vi "Test Selection.vi"() -> (0 "error out":errorcluster, 3 "Test Selected":string(combo))   [LabVIEW 2023, in "HardwareAbstractionLayer_LVOOP.lvlib" / "Report.lvclass"]
uses:
  Report.lvclass
panel:
  in  "Cancel":bool
  in  "Contionus Test":bool
  in  "New Test":bool
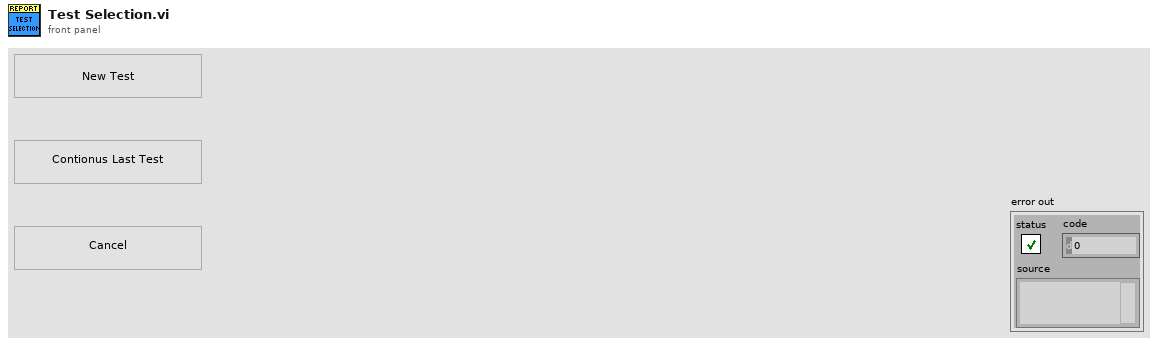
[diagram p1: front panel]
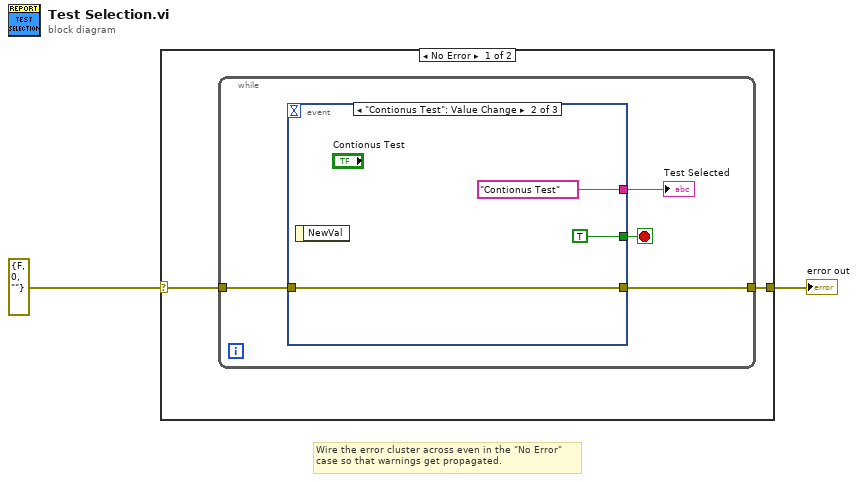
[diagram p0: block diagram]
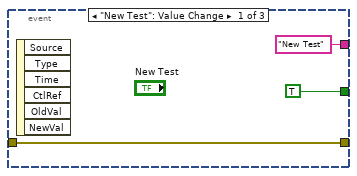
[diagram p2: hidden frame]
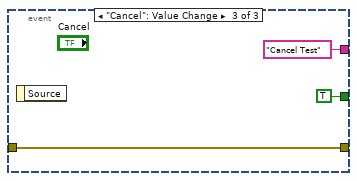
[diagram p3: hidden frame]
diagram:
  # "Wire the error cluster across even in the \"No Error\"\ncase so that warnings get propagated."
  n1 = case shown="No Error" errorcluster {"status"=FALSE, "code"=0, "source"=""} ("error in (no error)") {
    selector: errorcluster {"status"=FALSE, "code"=0, "source"=""} ("error in (no error)") -> [w4 w18]
    tunnel: [w3 w18] -> w2
    frame No Error {
      n2 = while {
        tunnel: w4 -> [w7]
        tunnel: [w6] -> w3
        stop <- w8 stop-if-true
        n3 = event shown="[1] \"Contionus Test\": Value Change" {
          selector: _ -> [_ _ _]
          dyn-events: _ -> [_ _ _]
          timeout: _ -> [_ _ _]
          tunnel: [TRUE TRUE TRUE] -> w8
          tunnel: w7 -> [w10 w13 w17]
          tunnel: [w10 w13 w17] -> w6
          tunnel: ["New Test" ("Test Selected") "Contionus Test" ("Test Selected") "Cancel Test" ("Test Selected")] -> w5
          event "New Test": Value Change {
            n4 = event-data() -> ()  [unwired: 1 in, 6 out]
          }
          event "Contionus Test": Value Change {
            n5 = event-data() -> ()  [unwired: 1 in, 1 out]
          }
          event "Cancel": Value Change {
            n6 = event-data() -> ()  [unwired: 1 in, 1 out]
          }
        }
        "Test Selected" <- w5
      }
    }
    frame Error {
    }
  }
  "error out" <- w2
